vi "SVT Octave Analysis [ANSI] (1 Ch).vi"(0 "scaled signal [EU]":waveform(dbl)={"t0"=timestamp(0 s since 1904-01-01), "dt"=1.953125e-05, "Y"=[]}, 1 "restart averaging (F)":bool, 2 "reset filter (F)":bool, 5 "frequency range":T8={"low band"=enum."16 Hz", "high band"=enum."16000 Hz"}, 9 "dB On (T)":bool=TRUE, 11 "error in (no error)":errorcluster, 12 "averaging type":T7(ring), 13 "exp avg settings":T1={" mode"=enum."Fast", "time constant [ms]"=125.0} {"time constant [ms]" format="%.2f"}, 14 "equal confidence level [dB]":dbl=125.0 format="%.2f") -> (3 "filter settled":bool, 4 "octave spectrum":T2 {"band power" format="%.2f"; "nominal frequencies [Hz]" format="%.2f"}, 6 "unit label":string, 8 "total band power":dbl format="%.2f", 10 "octave info":T3={"standard"=enum."ANSI S1.11", "bandwidth"=enum."1 octave", "low band"=0, "high band"=0, "weighting filter"=0, "dB reference"=0.0, "dB On"=FALSE, "unit label"="", "channel name"="", "description"="", "engineering units"=1, "custom label"="", "spectrum type"=enum."magnitude", "spectral density"=FALSE, "filters settled"=FALSE} {"engineering units" items=["custom..."=0, "V"=1, "A"=21, "C"=30, "pC"=31, "s"=32, "-"=29, "Pa"=2, "N"=20, "g"=3, "m/s^2"=4, "m/s"=5, "m"=6, "mm/s"=12, "mm"=13, "micron/s"=14, "micron"=15, "in/s^2"=7, "in/s"=8, "in"=9, "mil/s"=10, "mil"=11, "rad/s^2"=16, "rad/s"=17, "rad"=18, "deg/s^2"=26, "deg/s"=27, "deg"=28, "RPM"=22, "cycle/s^2"=23, "Hz"=24, "cycle"=25, "strain"=19]; "dB reference" format="%.2e"; "weighting filter" items=["Linear", "A-weighting", "B-weighting", "C-weighting", "ITU-R 468-4", "Dolby", "CCITT", "C-message", "Wb", "Wc", "Wd", "We", "Wf", "Wh", "Wj", "Wk", "Wm", "AES17 20 kHz lowpass", "AES17 40 kHz lowpass", "AES17 20 kHz highpass", "AES17 40 kHz highpass"]}, 15 "error out":errorcluster)   [LabVIEW 2017, in "SoundVib_Octave.lvlib"]
doc: "LabVIEW no longer supports this VI. The SVT Octave Analysis [ANSI] VI is available for compatibility with previous versions of the LabVIEW Sound and Vibration Toolkit. This VI offers compliance with the old ANSI S1.11-1986 standard. This standard has been superseded by the new ANSI S1.11-2004 standard. If you want to ensure compliance with the latter standard, use the SVT Octave Analysis VI found in this directory: <LabVIEW>\\vi.lib\\addons\\Sound and Vibration\\svt_Octave.\n\nPerforms an octave analysis on the <B>scaled signal [EU]</B> in according with the ANSI S1.11-1986 standard. The data type you wire to the <B>scaled signal [EU]</B> input determines the polymorphic instance to use."
uses:
  <vilib>/addons/Sound and Vibration/svt_Octave/SoundVib_Octave.lvlib
  <vilib>/addons/_NISVFA/_Shared subVIs/Controls/svc_Octave Info.ctl
  <vilib>/addons/_NISVFA/_Shared subVIs/Controls/svc_Octave Standard.ctl
  <vilib>/addons/_NISVFA/_Shared subVIs/Controls/svc_Weighting Filter Text Ring.ctl
  <vilib>/addons/_NISVFA/_Shared subVIs/Controls/svc_Engineering Units Text Ring.ctl
  <vilib>/addons/Sound and Vibration/svt_Octave_2014 standard/SoundVib_Octave_2014 standard.lvlib
panel:
  out "# samples to settle":u64
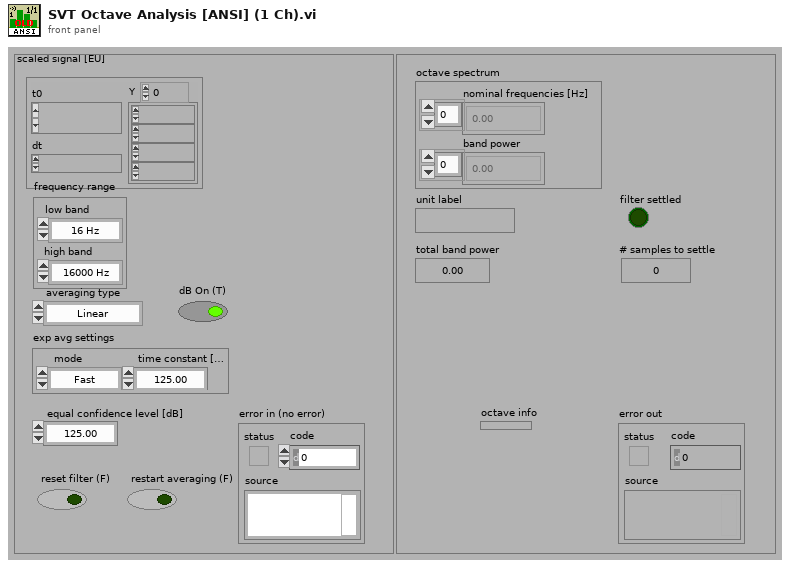
[diagram p1: front panel]
types:
  T1 = cluster{" mode":enum16{"Slow", "Fast", "Impulse", "Custom"}, "time constant [ms]":dbl}
  T2 = cluster{"nominal frequencies [Hz]":dbl[], "band power":dbl[]}
  T3 = typedef "svc_Octave Info.ctl" = cluster{"standard":T4, "bandwidth":enum16{"1 octave", "1/3 octave", "1/6 octave", "1/12 octave", "1/24 octave"}, "low band":i32, "high band":i32, "weighting filter":T5, "dB reference":dbl, "dB On":bool, "unit label":string, "channel name":string, "description":string, "engineering units":T6, "custom label":string, "spectrum type":enum16{"power", "magnitude"}, "spectral density":bool, "filters settled":bool}
  T4 = typedef "svc_Octave Standard.ctl" = enum16{"ANSI S1.11", "IEC 61260"}
  T5 = typedef "svc_Weighting Filter Text Ring.ctl" = u16
  T6 = typedef "svc_Engineering Units Text Ring.ctl" = u16
  T7 = enum16{"Linear", "Exponential", "Equal confidence", "Peak"}
  T8 = cluster{"low band":enum16{"16 Hz", "31.5 Hz", "63 Hz", "125 Hz", "250 Hz", "500 Hz", "1000 Hz", "2000 Hz", "4000 Hz", "8000 Hz", "16000 Hz"}, "high band":enum16{"16 Hz", "31.5 Hz", "63 Hz", "125 Hz", "250 Hz", "500 Hz", "1000 Hz", "2000 Hz", "4000 Hz", "8000 Hz", "16000 Hz"}}
  T9 = cluster{"standard":T4, "bandwidth":enum16{"1 octave", "1/3 octave", "1/6 octave", "1/12 octave", "1/24 octave"}}
  T10 = cluster{"nominal frequencies [Hz]":dbl[], "band power [EU^2 rms]":dbl[]}
  T11 = cluster{"nominal frequencies [Hz]":dbl[], "band power [dB EU]":dbl[]}
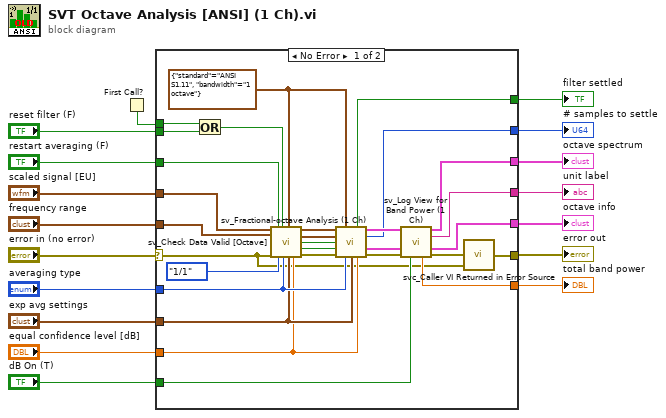
[diagram p0: block diagram]
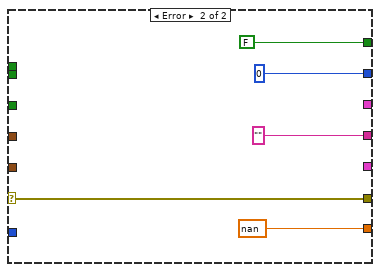
[diagram p2: hidden frame]
diagram:
  n1 = First Call?() -> (First Call?: T/F=w15:bool)
  n2 = case shown="No Error" "error in (no error)" {
    selector: "error in (no error)" -> [w18 w48]
    tunnel: "frequency range" -> [w46 _]
    tunnel: "reset filter (F)" -> [w20 _]
    tunnel: w15 -> [w19 _]
    tunnel: [w42 nan ("total band power [dB EU]")] -> w14
    tunnel: [w26 FALSE ("settled?")] -> w13
    tunnel: "restart averaging (F)" -> [w41 _]
    tunnel: "averaging type" -> [w39 _]
    tunnel: "exp avg settings" -> [w37 _]
    tunnel: "equal confidence level [dB]" -> [w24 _]
    tunnel: "dB On (T)" -> [w36 _]
    tunnel: [w33 _] -> w7
    tunnel: [w32 "" ("unit label")] -> w6
    tunnel: "scaled signal [EU]" -> [w31 _]
    tunnel: [w29 _] -> w4
    tunnel: [w28 w48] -> w3
    tunnel: [w21 u64 0 ("# samples to settle")] -> w1
    frame No Error {
      w27 = T9 {"standard"=enum."ANSI S1.11", "bandwidth"=enum."1 octave"} ("1/n Octave settings")
      n3 = Or(x=w19, y=w20) -> (x .or. y?=w23:bool)
      n4 = call <vilib>:"sv_Check Data Valid [Octave].vi"("scaled signal [EU]"=w31, "frequency range (1/1)"=w46, "error in (no error)"=w18, "restart averaging (F)"=w41, "bandwidth"=enum16{"1/1", "1/3", "1/n"}."1/1", "reset filter (F)"=w23, "averaging type"=w39, "1/n octave settings"=w27, "exp avg settings"=w37, "equal confidence level [dB]"=w24) -> ("dup scaled signal [EU]"=w44:waveform(dbl), "band number"=w35:cluster{"low band":i32, "high band":i32}, "Restart averaging"=w40:bool, "Reset Filter"=w25:bool, "error out"=w45:errorcluster)  [unwired: 5 in]
      n5 = call <vilib>:"sv_Fractional-octave Analysis (1 Ch).vi"("scaled signal [EU]"=w44, "1/n Octave settings"=w27, "band number"=w35, "restart averaging (F)"=w40, "reset filter (F)"=w25, "error in (no error)"=w45, "averaging type"=w39, "exp avg settings"=w37, "equal confidence level [dB]"=w24) -> ("settled?"=w26:bool, "octave spectrum"=w38:T10, "# samples to settle"=w21:u64, "octave info"=w30:T3, "error out"=w43:errorcluster)  [unwired: 2 in]
      n6 = call <vilib>:"sv_Log View for Band Power (1 Ch).vi"("octave spectrum"=w38, "octave info"=w30, "error in (no error)"=w43, "dB On (T)"=w36) -> ("octave spectrum"=w33:T11, "unit label"=w32:string, "octave info"=w29:T3, "total band power [dB EU]"=w42:dbl, "error out"=w34:errorcluster)  [unwired: 7 in]
      n7 = call <vilib>:"svc_Caller VI Returned in Error Source.vi"("warning input to caller"=w18, "error in (no error)"=w34) -> ("error out"=w28:errorcluster)  [unwired: 3 in]
    }
    frame Error {
    }
  }
  "filter settled" <- w13
  "unit label" <- w6
  "total band power" <- w14
  "error out" <- w3
  "octave info" <- w4
  "octave spectrum" <- w7
  "# samples to settle" <- w1
